vi "Release shared lock.vi"(8 "error in (no error)":errorcluster) -> (0 "error out":errorcluster, 1 "Safe to delete":bool)   [LabVIEW 2015, in "RefMem DMA Custom Device.lvlib"]
uses:
  RefMem DMA Custom Device.lvlib
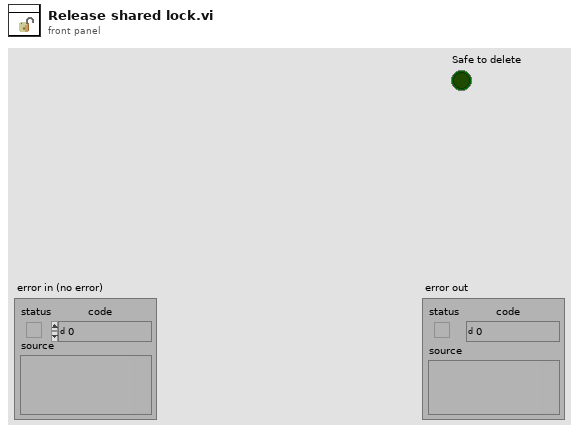
[diagram p1: front panel]
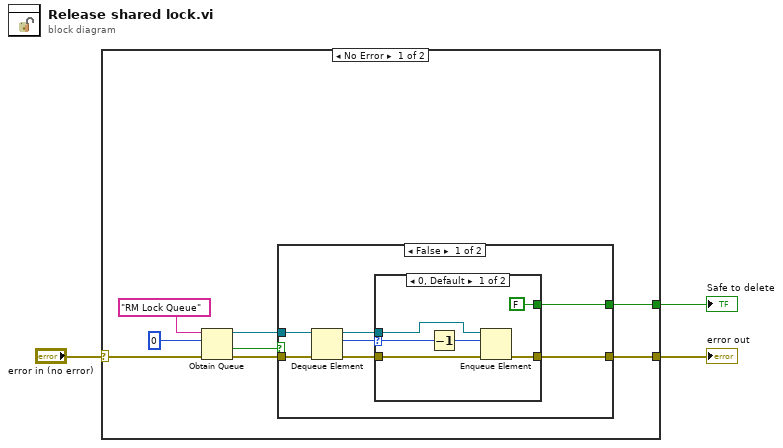
[diagram p0: block diagram]
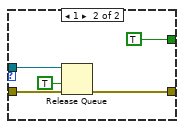
[diagram p2: hidden frame]
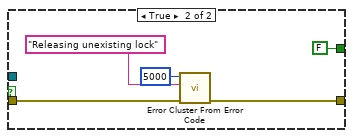
[diagram p3: hidden frame]
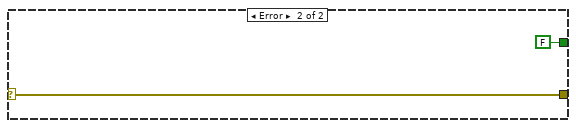
[diagram p4: hidden frame]
diagram:
  n1 = case shown="No Error" "error in (no error)" {
    selector: "error in (no error)" -> [w10 w36]
    tunnel: [w6 w36] -> w2
    tunnel: [w4 FALSE ("Safe to delete")] -> w1
    frame No Error {
      n2 = Obtain Queue(name (unnamed)="RM Lock Queue", element data type=0, error in (no error)=w10) -> (queue out=w8:refnum<queue>, created new?=w9:bool, error out=w7:errorcluster)  [unwired: 2 in]
      n3 = case shown="False" w9 {
        tunnel: w8 -> [w18 _]
        tunnel: w7 -> [w17 w34]
        tunnel: [w15 w33] -> w6
        tunnel: [w12 FALSE ("Safe to delete")] -> w4
        frame False {
          n4 = Dequeue Element(queue=w18, error in (no error)=w17) -> (queue out=w13:refnum<queue>, element=w14:i32, error out=w16:errorcluster)  [unwired: 1 in, 1 out]
          n5 = case shown="0, Default" w14 {
            selector: w14 -> [w19 _]
            tunnel: w16 -> [w24 w29]
            tunnel: [w22 w28] -> w15
            tunnel: w13 -> [w20 w27]
            tunnel: [FALSE ("Safe to delete") TRUE ("Safe to delete")] -> w12
            frame 0, Default {
              n6 = Decrement(x=w19) -> (x-1=w23:i32)
              n7 = Enqueue Element(queue=w20, element=w23, error in (no error)=w24) -> (error out=w22:errorcluster)  [unwired: 1 in, 2 out]
            }
            frame 1 {
              n8 = Release Queue(queue=w27, force destroy? (F)=TRUE, error in (no error)=w29) -> (error out=w28:errorcluster)  [unwired: 2 out]
            }
          }
        }
        frame True {
          n9 = call <vilib>:"Error Cluster From Error Code.vi"("error in (no error)"=w34, "error message (\"\")"="Releasing unexisting lock" ("error message (\"\")"), "error code (0)"=5000) -> ("error out"=w33:errorcluster)  [unwired: 6 in]
        }
      }
    }
    frame Error {
    }
  }
  "error out" <- w2
  "Safe to delete" <- w1
